vi "Sync DSA Instruments.vi"(0 "TSM context":T1) -> (15 "error out":errorcluster)   [LabVIEW 2020]
doc: "Sensitivity Test VI helps to source a known wavefrom (1k Hz) in speaker and capture back the waveform in the DUT and calculate the sensitivity in dBV"
uses:
  <vilib>/NI_TestStand_SemiconductorModule/NI_TestStand_Semiconductor_Module.lvlibp/PinMap/General/SemiconductorModuleContext.ctl
  580befc9-3443-43a1-ac84-b2f599be9b8b.vi
  580befc9-3443-43a1-ac84-b2f599be9b8b.vi/e325d36d-f8d5-444c-95fc-e56b98c083a2.vi
  <vilib>/NI_TestStand_SemiconductorModule/NI_TestStand_Semiconductor_Module.lvlibp
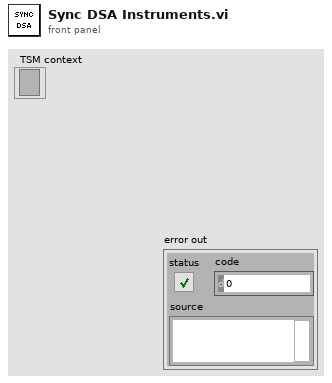
[diagram p1: front panel]
types:
  T1 = typedef "NI_TestStand_Semiconductor_Module.lvlibp/SemiconductorModuleContext.ctl" = refnum<k7>
  T2 = typedef "TSM DAQmx Multi-Task.ctl" = cluster{"Pin Query Context":refnum<class "MultiplePinMultipleSessionQueryContext.lvclass">, "SSC":T3[], "Site Numbers":i32[], "Pins":tag[]}
  T3 = typedef "SSC DAQmx.ctl" = cluster{"DAQmx Task ":refnum<k21>, "Channels":string, "Channel Lists":string}
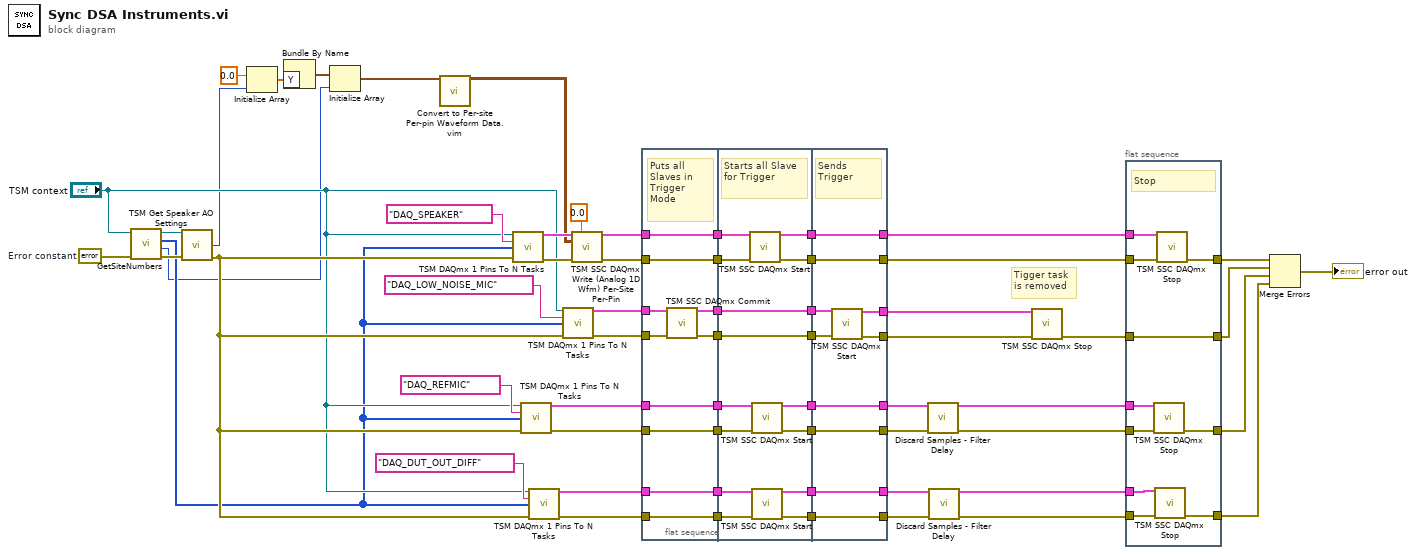
[diagram p0: block diagram]
diagram:
  w62 = errorcluster {"status"=FALSE, "code"=0, "source"=""}  # Error constant
  # "Tigger task \nis removed"
  n1 = call <vilib>:"GetSiteNumbers.vi"("error in (no error)"=w62, "Semiconductor Module Context"="TSM context") -> ("error out"=w42:errorcluster, "Number Of Sites"=w2:i32, "Site Numbers"=w17:i32[], "Semiconductor Module Context Out"=w41:T1)  [unwired: 6 in]
  n2 = call "TSM Get Speaker AO Settings.vi"("TSM context"=w41, "error in (no error)"=w42) -> ("Samples per channel"=w6:i32, "error out"=w43:errorcluster)  [unwired: 9 in, 3 out]
  n3 = Initialize Array(0.0 ("element"), w6) -> (w4:dbl[])
  n4 = Bundle By Name("Y"=w4) -> (w3:waveform(dbl))  [unwired: 1 in]
  n5 = Initialize Array(w3, w2) -> (w1:waveform(dbl)[])
  n6 = call "Convert to Per-site Per-pin Waveform Data.vim"("Waveform In"=w1) -> ("Per Site Per Pin Waveform Out"=w15:waveform(dbl)[][])  [unwired: 14 in]
  n7 = call "TSM DAQmx 1 Pins To N Tasks.vi"("TSM context"="TSM context", "Pins"=tag "DAQ_SPEAKER", "Site Numbers"=w17, "error in"=w43) -> ("DAQ TSM Out"=w56:T2, "error out"=w57:errorcluster)  [unwired: 10 in]
  n8 = call "TSM DAQmx 1 Pins To N Tasks.vi"("TSM context"="TSM context", "Pins"=tag "DAQ_REFMIC", "Site Numbers"=w17, "error in"=w43) -> ("DAQ TSM Out"=w49:T2, "error out"=w53:errorcluster)  [unwired: 10 in]
  n9 = call "TSM DAQmx 1 Pins To N Tasks.vi"("TSM context"="TSM context", "Pins"=tag "DAQ_DUT_OUT_DIFF", "Site Numbers"=w17, "error in"=w43) -> ("DAQ TSM Out"=w48:T2, "error out"=w52:errorcluster)  [unwired: 10 in]
  n10 = call "TSM DAQmx 1 Pins To N Tasks.vi"("TSM context"="TSM context", "Pins"=tag "DAQ_LOW_NOISE_MIC", "Site Numbers"=w17, "error in"=w43) -> ("DAQ TSM Out"=w22:T2, "error out"=w27:errorcluster)  [unwired: 10 in]
  n11 = call "TSM SSC DAQmx Write (Analog 1D Wfm) Per-Site Per-Pin.vi"("DAQ TSM in"=w56, "Idle Channel Value (0)"=0.0, "Per-Site Per-Pin Waveforms in"=w15, "error in"=w57) -> ("DAQ TSM Out"=w54:T2, "error out"=w55:errorcluster)  [unwired: 10 in]
  n12 = flat-sequence {
    tunnel: w48 -> [w67]
    tunnel: w49 -> [w68]
    tunnel: w54 -> [w69]
    tunnel: w55 -> [w70]
    tunnel: w52 -> [w71]
    tunnel: w53 -> [w72]
    tunnel: [w72] -> w40
    tunnel: [w71] -> w39
    tunnel: [w70] -> w38
    tunnel: [w69] -> w37
    tunnel: [w68] -> w36
    tunnel: [w67] -> w35
    tunnel: w27 -> [w66]
    tunnel: [w65] -> w26
    tunnel: w22 -> [w64]
    tunnel: [w63] -> w20
    tunnel: w40 -> [w86]
    tunnel: w39 -> [w85]
    tunnel: w38 -> [w76]
    tunnel: w37 -> [w74]
    tunnel: w36 -> [w82]
    tunnel: w35 -> [w81]
    tunnel: [w75] -> w34
    tunnel: [w73] -> w33
    tunnel: [w84] -> w32
    tunnel: [w83] -> w31
    tunnel: [w80] -> w30
    tunnel: [w79] -> w29
    tunnel: w26 -> [w78]
    tunnel: [w78] -> w25
    tunnel: [w77] -> w21
    tunnel: w20 -> [w77]
    tunnel: [w91] -> w12
    tunnel: [w92] -> w8
    tunnel: [w93] -> w14
    tunnel: [w94] -> w10
    tunnel: [w95] -> w50
    tunnel: [w96] -> w51
    tunnel: w34 -> [w96]
    tunnel: w33 -> [w95]
    tunnel: w32 -> [w94]
    tunnel: w31 -> [w93]
    tunnel: w30 -> [w92]
    tunnel: w29 -> [w91]
    tunnel: w25 -> [w90]
    tunnel: [w89] -> w24
    tunnel: w21 -> [w88]
    tunnel: [w87] -> w19
    frame #0 {
      # "Puts all Slaves in Trigger Mode"
      n13 = call "TSM SSC DAQmx Commit.vi"("TSM DAQmx In"=w64, "error in (no error)"=w66) -> ("TSM DAQmx Out"=w63:T2, "error out"=w65:errorcluster)  [unwired: 12 in]
    }
    frame #1 {
      # "Starts all Slave for Trigger"
      n14 = call "TSM SSC DAQmx Start.vi"("TSM DAQmx In"=w74, "error in (no error)"=w76) -> ("TSM DAQmx Out"=w73:T2, "error out"=w75:errorcluster)  [unwired: 12 in]
      n15 = call "TSM SSC DAQmx Start.vi"("TSM DAQmx In"=w82, "error in (no error)"=w86) -> ("TSM DAQmx Out"=w80:T2, "error out"=w84:errorcluster)  [unwired: 12 in]
      n16 = call "TSM SSC DAQmx Start.vi"("TSM DAQmx In"=w81, "error in (no error)"=w85) -> ("TSM DAQmx Out"=w79:T2, "error out"=w83:errorcluster)  [unwired: 12 in]
    }
    frame #2 {
      # "Sends Trigger"
      n17 = call "TSM SSC DAQmx Start.vi"("TSM DAQmx In"=w88, "error in (no error)"=w90) -> ("TSM DAQmx Out"=w87:T2, "error out"=w89:errorcluster)  [unwired: 12 in]
    }
  }
  n18 = call "Discard Samples - Filter Delay.vi"("DAQ TSM in"=w8, "error in"=w10) -> ("DAQ TSM Out"=w7:T2, "error out"=w9:errorcluster)  [unwired: 12 in]
  n19 = call "Discard Samples - Filter Delay.vi"("DAQ TSM in"=w12, "error in"=w14) -> ("DAQ TSM Out"=w11:T2, "error out"=w13:errorcluster)  [unwired: 12 in]
  n20 = call "TSM SSC DAQmx Stop.vi"("TSM DAQmx In"=w19, "error in (no error)"=w24) -> ("error out"=w23:errorcluster)  [unwired: 12 in, 1 out]
  n21 = flat-sequence {
    tunnel: w51 -> [w106]
    tunnel: [w105] -> w47
    tunnel: w50 -> [w104]
    tunnel: w9 -> [w103]
    tunnel: [w102] -> w46
    tunnel: w13 -> [w101]
    tunnel: [w100] -> w45
    tunnel: w11 -> [w99]
    tunnel: w7 -> [w98]
    tunnel: w23 -> [w97]
    tunnel: [w97] -> w16
    frame #0 {
      # "Stop"
      n22 = call "TSM SSC DAQmx Stop.vi"("TSM DAQmx In"=w98, "error in (no error)"=w103) -> ("error out"=w102:errorcluster)  [unwired: 12 in, 1 out]
      n23 = call "TSM SSC DAQmx Stop.vi"("TSM DAQmx In"=w99, "error in (no error)"=w101) -> ("error out"=w100:errorcluster)  [unwired: 12 in, 1 out]
      n24 = call "TSM SSC DAQmx Stop.vi"("TSM DAQmx In"=w104, "error in (no error)"=w106) -> ("error out"=w105:errorcluster)  [unwired: 12 in, 1 out]
    }
  }
  n25 = Merge Errors(w47, w16, w46, w45) -> (→"error out":errorcluster)
